vi "Run Bfr Tx - Sim Buffer Data.vi"(8 "error in (no error)":errorcluster, 11 "Tx Loop Data in":T1 {"Data Buffer" format="%016x"}) -> (0 "error out":errorcluster, 3 "Tx Loop Data out":T1 {"Data Buffer" format="%016x"})   [LabVIEW 2016, in "UDP-Custom-Device Engine.lvlib"]
uses:
  UDP-Custom-Device Engine.lvlib
  Types/Engine - Buffered Tx Loop Data.ctl
  Shared/Types/Shared - Header Details.ctl
  Shared/Types/Shared - Buffered.PacketInfo.ctl
  Shared/Types/Shared - Pointer Encoding.ctl
  <vilib>/NI/NIVS Inline Async API/_Data Access Engine/Data Access Engine/Types/ReadWrite.DVR.ctl
  <vilib>/NI/NIVS Inline Async API/_Data Access Engine/Access Type Classes/ReadWrite/ReadWrite.lvclass
  <vilib>/NI/NIVS Inline Async API/_Data Access Engine/Data Access Engine/Types/Read.DVR.ctl
  <vilib>/NI/NIVS Inline Async API/_Data Access Engine/Access Type Classes/Read/Read.lvclass
  <vilib>/NI/NIVS Inline Async API/_Data Access Engine/Data Access Engine/Types/Write.DVR.ctl
  <vilib>/NI/NIVS Inline Async API/_Data Access Engine/Access Type Classes/Write/Write.lvclass
  Shared/Types/Shared - Duplex Settings.ctl
  <vilib>/NI Veristand/VeriStand Data/Library/Pointer Operations/Pointer.Write (String).vi
  <vilib>/NI Veristand/VeriStand Data/Library/Pointer Operations/Pointer.Write (1D U8).vi
  <vilib>/NI Veristand/VeriStand Data/Library/VeriStand Data.lvlib
  Shared/UDP-Custom-Device Shared.lvlib
  <vilib>/NI/NIVS Inline Async API/_Data Access Engine/Data Access Engine/Data Access Engine.lvclass
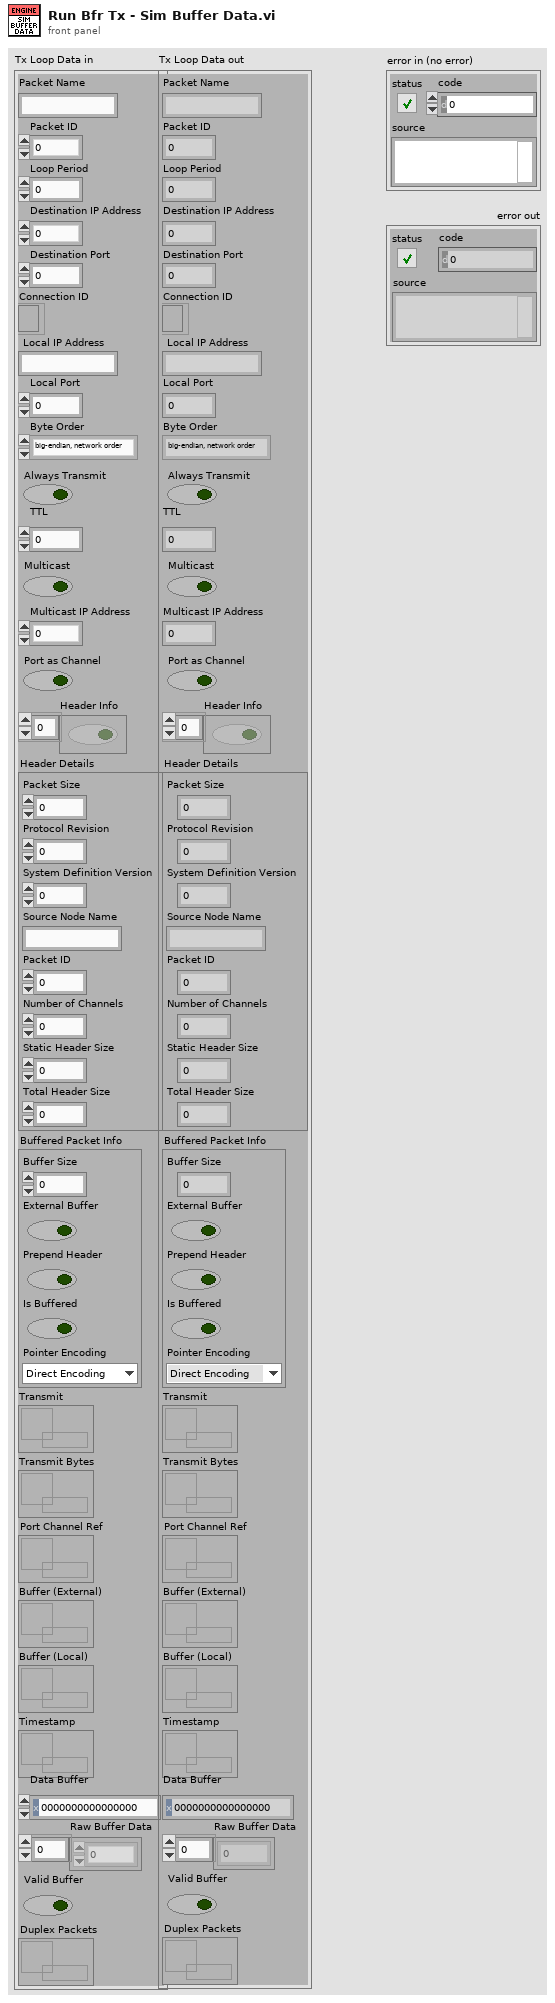
[diagram p1: front panel]
types:
  T1 = typedef "UDP-Custom-Device Engine.lvlib/Engine - Buffered Tx Loop Data.ctl" = cluster{"Packet Name":string, "Packet ID":i32, "Loop Period":u32, "Destination IP Address":u32, "Destination Port":u16, "Connection ID":refnum<k16>, "Local IP Address":string, "Local Port":i32, "Byte Order":enum16{"big-endian, network order", "native, host order", "little-endian"}, "Always Transmit":bool, "TTL":u16, "Multicast":bool, "Multicast IP Address":u32, "Port as Channel":bool, "Header Info":bool[], "Header Details":T2, "Buffered Packet Info":T3, "Transmit":T5, "Transmit Bytes":T6, "Port Channel Ref":T6, "Buffer (External)":T6, "Buffer (Local)":T7, "Timestamp":T6, "Data Buffer":u64, "Raw Buffer Data":u8[], "Valid Buffer":bool, "Duplex Packets":refnum<data-value>}
  T2 = typedef "UDP-Custom-Device Shared.lvlib/Shared - Header Details.ctl" = cluster{"Packet Size":u16, "Protocol Revision":u8, "System Definition Version":u64, "Source Node Name":string, "Packet ID":u32, "Number of Channels":u32, "Static Header Size":u16, "Total Header Size":u16}
  T3 = typedef "UDP-Custom-Device Shared.lvlib/Shared - Buffered.PacketInfo.ctl" = cluster{"Buffer Size":i32, "External Buffer":bool, "Prepend Header":bool, "Is Buffered":bool, "Pointer Encoding":T4}
  T4 = typedef "UDP-Custom-Device Shared.lvlib/Shared - Pointer Encoding.ctl" = enum16{"Direct Encoding", "Conversion Encoding"}
  T5 = typedef "Data Access Engine.lvlib/Data Access Engine.lvclass/ReadWrite.DVR.ctl" = refnum<data-value>
  T6 = typedef "Data Access Engine.lvlib/Data Access Engine.lvclass/Read.DVR.ctl" = refnum<data-value>
  T7 = typedef "Data Access Engine.lvlib/Data Access Engine.lvclass/Write.DVR.ctl" = refnum<data-value>
  T8 = enum16{"Counter", "FullBuffer", "NoSim", "Zero Blobs"}
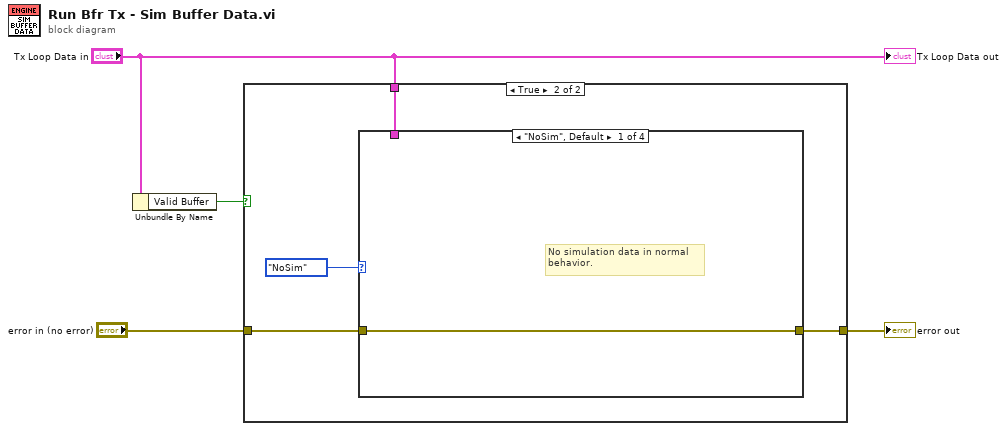
[diagram p0: block diagram]
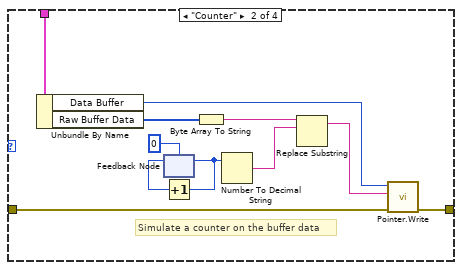
[diagram p3: hidden frame]
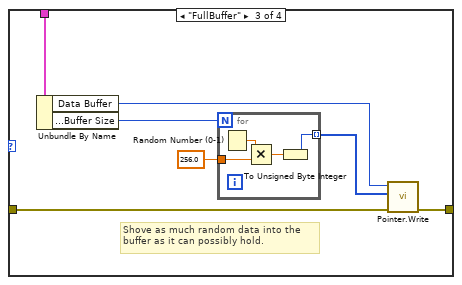
[diagram p4: hidden frame]
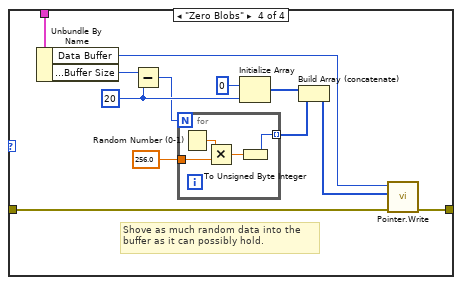
[diagram p5: hidden frame]
diagram:
  n1 = Unbundle By Name("Tx Loop Data in") -> ("Valid Buffer"=w1:bool)
  n2 = case shown="True" w1 {
    tunnel: "error in (no error)" -> [w5 w9]
    tunnel: [w5 w8] -> w3
    tunnel: "Tx Loop Data in" -> [_ w6]
    frame False {
    }
    frame True {
      n3 = case shown="\"NoSim\", Default" T8."NoSim" {
        tunnel: w6 -> [_ w21 w28 w44]
        tunnel: w9 -> [w10 w19 w26 w42]
        tunnel: [w10 w14 w25 w41] -> w8
        frame "NoSim", Default {
          # "No simulation data in normal\nbehavior."
        }
        frame "Counter" {
          # "Simulate a counter on the buffer data"
          n4 = Unbundle By Name(w21) -> ("Data Buffer"=w20:u64, "Raw Buffer Data"=w12:u8[])
          n5 = feedback #1(0) -> (w17:i32)
          n6 = Increment(x=w17) -> (x+1=w16:i32)
          n7 = feedback-in #1(w16) -> ()
          n8 = Byte Array To String(unsigned byte array=w12) -> (string=w11:string)
          n9 = Number To Decimal String(number=w16) -> (decimal integer string=w15:string)  [unwired: 1 in]
          n10 = Replace Substring(4:w15, 5:w11) -> (1:w13:string)  [unwired: 2 in, 1 out]
          n11 = call-poly <vilib>:"Pointer.Write.vi"("error in (no error)"=w19, "string in"=w13, "pointer in"=w20) -> ("error out"=w14:errorcluster)  [unwired: 6 in, 2 out]
        }
        frame "FullBuffer" {
          # "Shove as much random data into the\nbuffer as it can possibly hold."
          n12 = Unbundle By Name(w28) -> ("Data Buffer"=w27:u64, "Buffered Packet Info.Buffer Size"=w24:i32)
          n13 = for {
            N: w24 -> [_]
            tunnel: [w29] -> w22 mode=indexing
            tunnel: 256.0 -> [w31]
            n14 = Random Number (0-1)() -> (number: 0 to 1=w32:dbl)
            n15 = Multiply(x=w32, y=w31) -> (x*y=w30:dbl)
            n16 = To Unsigned Byte Integer(number=w30) -> (unsigned 8bit integer=w29:u8)
          }
          n17 = call-poly <vilib>:"Pointer.Write.vi"("error in (no error)"=w26, "values"=w22, "pointer in"=w27) -> ("error out"=w25:errorcluster)  [unwired: 6 in, 2 out]
        }
        frame "Zero Blobs" {
          w37 = 20 ("y")
          # "Shove as much random data into the\nbuffer as it can possibly hold."
          n18 = Unbundle By Name(w44) -> ("Data Buffer"=w43:u64, "Buffered Packet Info.Buffer Size"=w38:i32)
          n19 = Subtract(x=w38, y=w37) -> (x-y=w36:i32)
          n20 = for {
            N: w36 -> [_]
            tunnel: [w45] -> w34 mode=indexing
            tunnel: 256.0 -> [w47]
            n21 = Random Number (0-1)() -> (number: 0 to 1=w48:dbl)
            n22 = Multiply(x=w48, y=w47) -> (x*y=w46:dbl)
            n23 = To Unsigned Byte Integer(number=w46) -> (unsigned 8bit integer=w45:u8)
          }
          n24 = Initialize Array(u8 0, w37) -> (w35:u8[])
          n25 = Build Array (concatenate)(w35, w34) -> (w33:u8[])
          n26 = call-poly <vilib>:"Pointer.Write.vi"("error in (no error)"=w42, "values"=w33, "pointer in"=w43) -> ("error out"=w41:errorcluster)  [unwired: 6 in, 2 out]
        }
      }
    }
  }
  "error out" <- w3
  "Tx Loop Data out" <- "Tx Loop Data in"
